vi "Crawl_Folders.vi"(11 "path in":path[](array[path])) -> (1 "FileNames":string[](array[string]), 2 "Folders":path[](array[path]))   [LabVIEW 2018]
panel:
  out "error out":errorcluster
  in  "error in":errorcluster
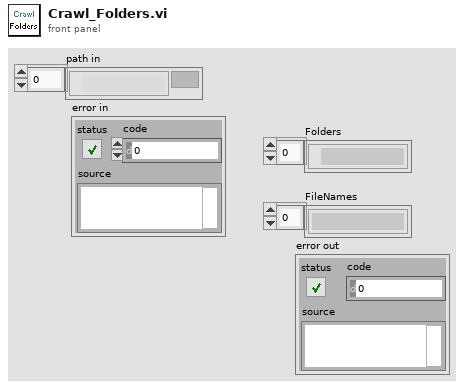
[diagram p1: front panel]
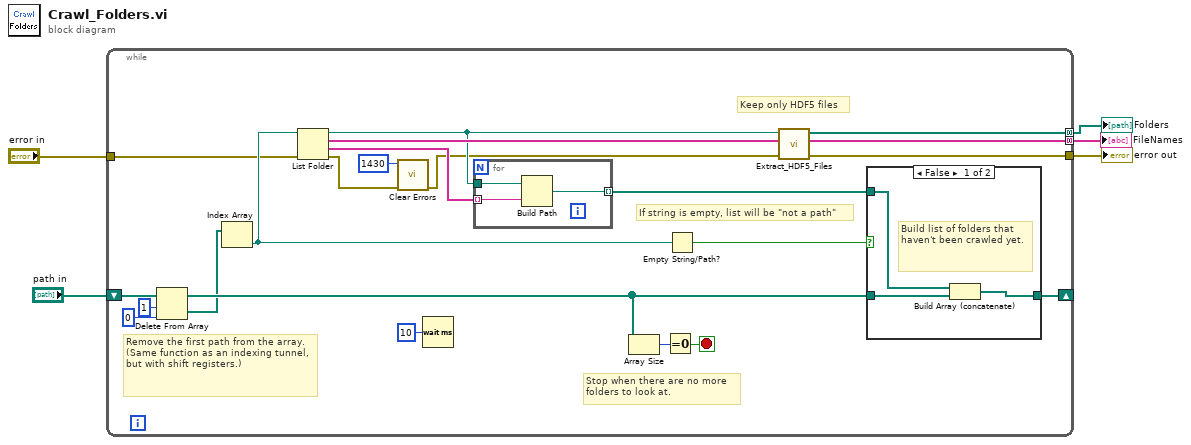
[diagram p0: block diagram]
diagram:
  n1 = while {
    shift-right: [w9] -> _
    shift-left: "path in" -> [w16]
    tunnel: [w24] -> w4 mode=concatenating
    tunnel: [w23] -> w5 mode=concatenating
    tunnel: "error in" -> [w8]
    tunnel: [w7] -> w1
    stop <- w18 stop-if-true
    # "Keep only HDF5 files"
    # "Remove the first path from the array. (Same function as an indexing tunnel, but with shift registers.)"
    # "Stop when there are no more\nfolders to look at."
    # "If string is empty, list will be \"not a path\""
    n2 = Delete From Array(array=w16, length=1, index=0) -> (deleted portion=w15:path[], array with subset deleted=w19:path[])
    n3 = Index Array(array=w15) -> (element=w14:path)  [unwired: 1 in]
    n4 = List Folder(path=w14, error in=w8) -> (path out=w12:path, filenames=w26:string[], folder names=w11:string[], error out=w21:errorcluster)  [unwired: 2 in]
    n5 = call <vilib>:"Clear Errors.vi"("error in (no error)"=w21, "specific error code to clear (0: all)"=1430) -> ("error out"=w7:errorcluster)  [unwired: 4 in, 1 out]
    n6 = Wait (ms)(milliseconds to wait=u32 10) -> ()  [unwired: 1 out]
    n7 = for {
      tunnel: w11 -> [w28] mode=indexing
      tunnel: w12 -> [w29]
      tunnel: [w27] -> w10 mode=indexing
      n8 = Build Path(base path=w29, name or relative path=w28) -> (appended path=w27:path)
    }
    n9 = Array Size(array=w19) -> (size(s)=w17:i32)
    n10 = Equal To 0?(x=w17) -> (x = 0?=w18:bool)
    n11 = Empty String/Path?(string/path=w14) -> (empty?=w13:bool)
    n12 = call "Extract_HDF5_Files.vi"("filenames"=w26, "path"=w12) -> ("FileNames"=w24:string[], "Folders"=w23:path[])  [unwired: 8 in]
    n13 = case shown="False" w13 {
      tunnel: w10 -> [w32 _]
      tunnel: w19 -> [w31 w33]
      tunnel: [w30 w33] -> w9
      frame False {
        # "Build list of folders that haven't been crawled yet."
        n14 = Build Array (concatenate)(w32, w31) -> (w30:path[])
      }
      frame True {
      }
    }
  }
  "Folders" <- w5
  "FileNames" <- w4
  "error out" <- w1
